vi "Compute DistanceToBalls.vi"(6 "Target Width (in)":dbl=6.0 format="%#_13g", 7 "Interpolation Table":dbl[][](array[numeric])=[[60.0, 133.0, 177.0, 222.0]] format="%0.2f", 8 "results":T1, 10 "FOV":dbl=41.0, 11 "Image Src":T2) -> (0 "results out":T1, 1 "Off Angle":dbl, 2 "Raw Ball DIstance":dbl, 3 "Image Dst Out":T2)   [LabVIEW 2019]
doc: "Using the camera lens information and the real world size of the target, use trig and ratios to determine the distance to the target. Also returns the location relative to the image center in a (-1 , 1) coordinate system that may be useful for steering the robot."
uses:
  <vilib>/vision/Image Controls.llb/IMAQ Image.ctl
  Vision Support Code/Target Fields.ctl
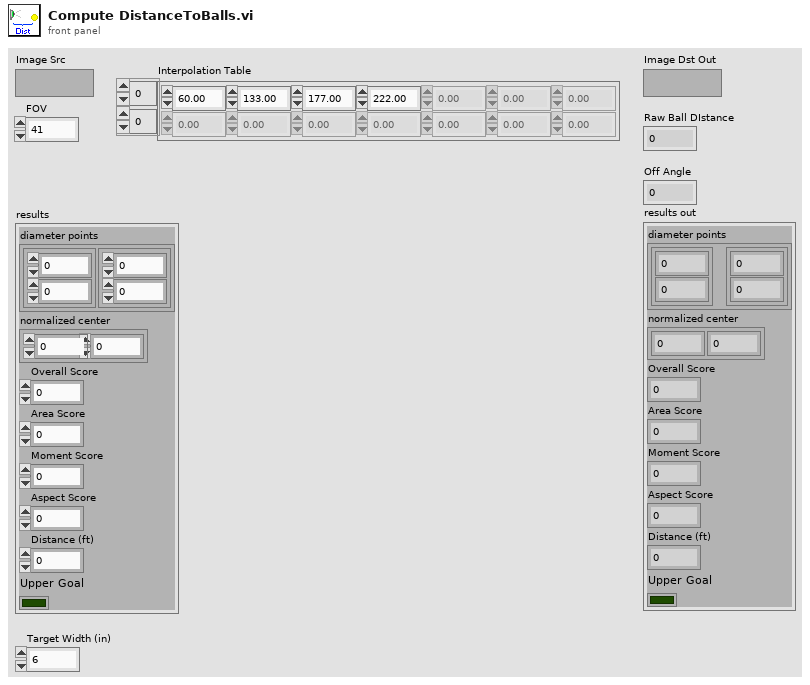
[diagram p1: front panel]
types:
  T1 = typedef "Target Fields.ctl" = cluster{"diameter points":cluster{"first point":cluster{"x":dbl, "y":dbl}, "projected point":cluster{"x":dbl, "y":dbl}}, "normalized center":cluster{"x":dbl, "y":dbl}, "Overall Score":dbl, "Area Score":dbl, "Moment Score":dbl, "Aspect Score":dbl, "Distance (ft)":dbl, "Upper Goal":bool}
  T2 = typedef "IMAQ Image.ctl" = refnum<image>
  T3 = cluster{"first point":cluster{"x":dbl, "y":dbl}, "projected point":cluster{"x":dbl, "y":dbl}}
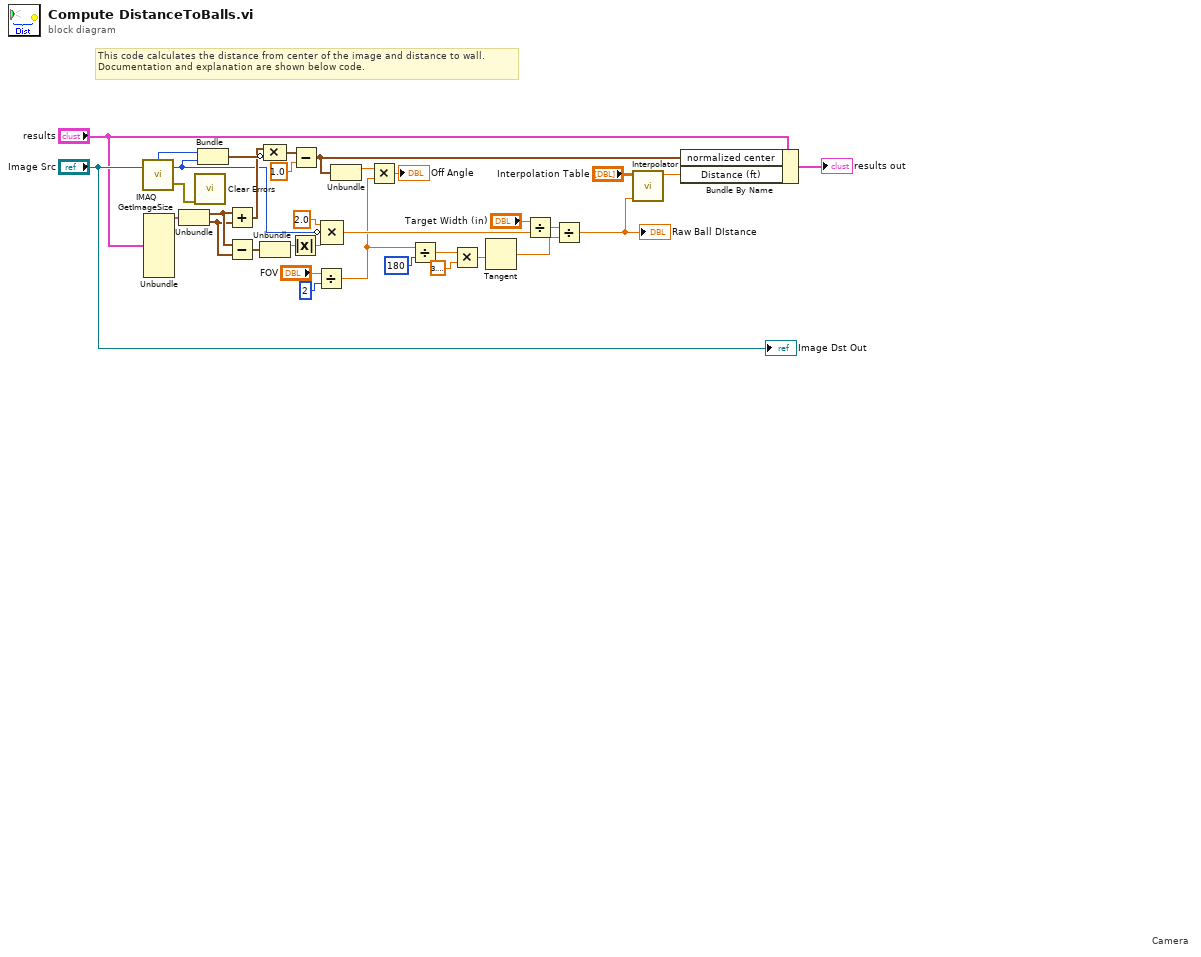
[diagram p0: block diagram]
diagram:
  # "Camera"
  # "This code calculates the distance from center of the image and distance to wall.\nDocumentation and explanation are shown below code."
  n1 = call "IMAQ GetImageSize"("Image"="Image Src") -> ("Y Resolution"=w12:i32, "X Resolution"=w9:i32, "error out"=w26:errorcluster)  [unwired: 3 in]
  n2 = Unbundle("results") -> ("diameter points"=w19:T3)  [unwired: 7 out]
  n3 = Unbundle(w19) -> ("first point"=w16:cluster{"x":dbl, "y":dbl}, "projected point"=w15:cluster{"x":dbl, "y":dbl})
  n4 = call <vilib>:"Clear Errors.vi"("error in (no error)"=w26) -> ()  [unwired: 5 in, 2 out]
  n5 = Bundle("X Resolution"=w9, "Y Resolution"=w12) -> (w17:cluster{"X Resolution":i32, "Y Resolution":i32})  [unwired: 1 in]
  n6 = Add(x=w16, y=w15) -> (x+y=w14:cluster{"x":dbl, "y":dbl})
  n7 = Subtract(x=w16, y=w15) -> (x-y=w23:cluster{"x":dbl, "y":dbl})
  n8 = Unbundle(w23) -> ("x"=w22:dbl)  [unwired: 1 out]
  n9 = Compound Arithmetic op=MULTIPLY(w14, invert w17) -> (w18:cluster{dbl, dbl})
  n10 = Absolute Value(x=w22) -> (abs(x)=w24:dbl)
  n11 = Subtract(x=w18, y=1.0) -> (x-y=w10:cluster{dbl, dbl})
  n12 = Divide(x="FOV", y=2) -> (x/y=w4:dbl)
  n13 = Compound Arithmetic op=MULTIPLY(2.0, invert w12, w24) -> (w27:dbl)
  n14 = Unbundle(w10) -> (w7:dbl)  [unwired: 1 out]
  n15 = Multiply(x=w7, y=w4) -> (x*y=→"Off Angle":dbl)
  n16 = Divide(x=w4, y=180) -> (x/y=w31:dbl)
  n17 = Multiply(x=w31, y=3.141592653589793) -> (x*y=w32:dbl)
  n18 = Tangent(1:w32) -> (0:w29:dbl)
  n19 = Divide(x="Target Width (in)", y=w27) -> (x/y=w6:dbl)
  n20 = Divide(x=w6, y=w29) -> (x/y=w2:dbl)
  "Raw Ball DIstance" <- w2
  n21 = call "Interpolator.vi"("Current Distance (ft)"=w2, "Interpolation Table"="Interpolation Table") -> ("Corrected DIstance"=w3:dbl)  [unwired: 9 in]
  n22 = Bundle By Name(cluster="results", "normalized center"=w10, "Distance (ft)"=w3) -> (→"results out":T1)
  "Image Dst Out" <- "Image Src"
